vi "Gain Set.vi"(8 "error in (no error)":errorcluster, 10 "Gain":u8 step=1, 11 "Camera_Controller in":refnum<class "Camera_Controller.lvclass">) -> (0 "error out":errorcluster, 3 "Camera_Controller out":refnum<class "Camera_Controller.lvclass">)   [LabVIEW 2023, in "Camera_Controller.lvlib" / "Camera_Controller.lvclass"]
uses:
  Camera_Controller.lvclass
  Camera_Controller.lvclass/Camera_Controller.ctl
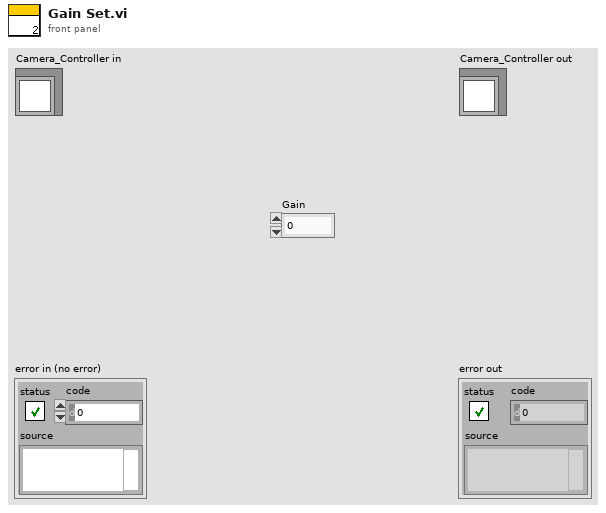
[diagram p1: front panel]
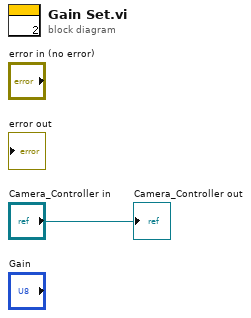
[diagram p0: block diagram]
diagram:
  "Camera_Controller out" <- "Camera_Controller in"
